vi "Finish.vi"   [LabVIEW 2012]
doc: "This VI is called just before exiting. It is expected to close I/O refnum, save collected data, etc."
uses:
  <vilib>/Rock Robotics/WPI/Compressor/WPI_CompressorGetSetRefNum.vi
  <vilib>/Rock Robotics/WPI/Joystick/WPI_JoystickGetSetRefNum.vi
  <vilib>/Rock Robotics/WPI/RobotDrive/WPI_RobotDriveGetSetRefNum.vi
types:
  T1 = typedef "WPI_JoystickDevRef.ctl" = cluster{"Device":T2}
  T2 = typedef "WPI_JoystickDeviceEnum.ctl" = enum16{"USB 1", "USB 2", "USB 3", "USB 4", "Kinect 1", "Kinect 2"}
  T3 = typedef "WPI_RobotDriveDevRef.ctl" = cluster{"DevStatus":errorcluster, "Motors[]":T4[], "Square Inputs":bool, "Max Output":dbl, "Isochronous":bool}
  T4 = typedef "WPI_MotorControlDeviceRef.ctl" = cluster{"DeviceStatus":errorcluster, "Type":enum16{"PWM", "CAN"}, "PWM":cluster{"Digital Module":T5, "PWM Channel":T6, "DeadBand":T7}, "CAN":cluster{"Device Number":u8, "Control Mode":T8, "Semaphore":T9, "Max Vout":dbl}, "Invert":bool, "TransformRef":T10, "InvTransformRef":T10}
  T5 = typedef "FPGA_TypedefDigitalModule.ctl" = enum16{"Digital Module 1", "Digital Module 2"}
  T6 = typedef "FPGA_DIOPWMChannel.ctl" = enum8{"PWM 1", "PWM 2", "PWM 3", "PWM 4", "PWM 5", "PWM 6", "PWM 7", "PWM 8", "PWM 9", "PWM 10", "Invalid"}
  T7 = typedef "WPI_PWMDeadband.ctl" = cluster{"Name":string, "maxPositivePwm":i32, "minPositivePwm":i32, "centerPwm":i32, "maxNegativePwm":i32, "minNegativePwm":i32, "angularRange":u16}
  T8 = typedef "WPI_CANJaguar_ControlMode.ctl" = enum8{"Percent VBus", "Current", "Speed", "Position", "Voltage"}
  T9 = typedef "Semaphore RefNum" = refnum<k1>
  T10 = typedef "WPI_PWMTransform_ConPane.ctl" = refnum<vi>
  T11 = typedef "WPI_CameraDevRef.ctl" = cluster{"Camera Address":string, "CameraStatus":errorcluster, "Acquire Image Notifier":refnum<notifier>}
  T12 = typedef "WPI_DigitalInputDevRef.ctl" = cluster{"DevStatus":errorcluster, "DIO Channel":T13, "Digital Module":T5}
  T13 = typedef "FPGA_DIOChannel.ctl" = enum8{"DIO 1", "DIO 2", "DIO 3", "DIO 4", "DIO 5", "DIO 6", "DIO 7", "DIO 8", "DIO 9", "DIO 10", "DIO 11", "DIO 12", "DIO 13", "DIO 14", "Invalid"}
  T14 = typedef "WPI_SolenoidDevRef.ctl" = cluster{"DevStatus":errorcluster, "Solenoid Module":T15, "Forward Solenoid Channel":T16, "Reverse Solenoid Channel":T16}
  T15 = typedef "FPGA_TypedefSolenoidModule.ctl" = enum16{"Solenoid Module 1", "Solenoid Module 2"}
  T16 = typedef "WPI_SolenoidChannel.ctl" = enum8{"Solenoid 1", "Solenoid 2", "Solenoid 3", "Solenoid 4", "Solenoid 5", "Solenoid 6", "Solenoid 7", "Solenoid 8", "Invalid"}
  T17 = typedef "WPI_CompressorDevRef.ctl" = cluster{"DevStatus":errorcluster, "DigitalInputDevRef":T12, "RelayDevRef":T18}
  T18 = typedef "WPI_RelayDevRef.ctl" = cluster{"DevStatus":errorcluster, "Relay Channel":T19, "Digital Module":T5, "Relay Direction":T20}
  T19 = typedef "FPGA_DIORelayChannel.ctl" = enum8{"Relay 1", "Relay 2", "Relay 3", "Relay 4", "Relay 5", "Relay 6", "Relay 7", "Relay 8", "Invalid"}
  T20 = typedef "WPI_RelayDirection.ctl" = enum16{"Both directions", "Forward only", "Reverse only"}
  T21 = typedef "WPI_EncoderDevRef.ctl" = cluster{"DevStatus":errorcluster, "EncoderIndex":T22, "CounterIndex":T23, "DistancePerCount":dbl, "Decoding Type":T24}
  T22 = typedef "FPGA_EncoderIdx.ctl" = enum8{"Enc 0", "Enc 1", "Enc 2", "Enc 3", "Invalid"}
  T23 = typedef "FPGA_CounterCtrSystemIndex.ctl" = enum8{"Ctr 0", "Ctr 1", "Ctr 2", "Ctr 3", "Ctr 4", "Ctr 5", "Ctr 6", "Ctr 7", "Invalid"}
  T24 = typedef "WPI_EncoderType.ctl" = enum16{"1x", "2x", "4x"}
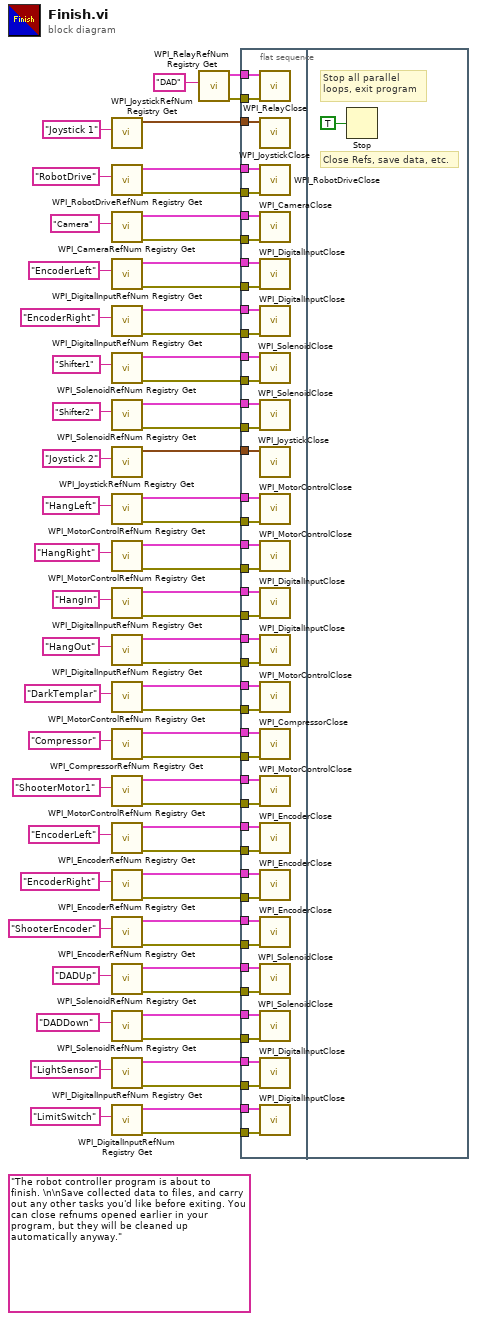
[diagram p0: block diagram]
diagram:
  (unwired) "The robot controller program is about to finish. \n\nSave collected data to files, and carry out any other tasks you'd like before exiting. You can close refnums opened earlier in your program, but they will be cleaned up automatically anyway."
  n1 = call <vilib>:"WPI_JoystickRefNum Registry Get.vi"("refnum name"="Joystick 1") -> ("JoystickDevRef"=w64:T1)  [unwired: 1 in, 9 out]
  n2 = call <vilib>:"WPI_RobotDriveRefNum Registry Get.vi"("refnum name"="RobotDrive") -> ("error out"=w61:errorcluster, "RobotDriveDevRef"=w65:T3)  [unwired: 1 in, 8 out]
  n3 = call <vilib>:"WPI_CameraRefNum Registry Get.vi"("refnum name"="Camera") -> ("error out"=w60:errorcluster, "CameraDevRef"=w63:T11)  [unwired: 1 in, 8 out]
  n4 = call <vilib>:"WPI_DigitalInputRefNum Registry Get.vi"("refnum name"="EncoderLeft") -> ("error out"=w54:errorcluster, "DigitalInputDevRef"=w55:T12)  [unwired: 9 in]
  n5 = call <vilib>:"WPI_DigitalInputRefNum Registry Get.vi"("refnum name"="EncoderRight") -> ("error out"=w53:errorcluster, "DigitalInputDevRef"=w48:T12)  [unwired: 9 in]
  n6 = call <vilib>:"WPI_SolenoidRefNum Registry Get.vi"("refnum name"="Shifter1") -> ("error out"=w51:errorcluster, "SolenoidDevRef"=w52:T14)  [unwired: 9 in]
  n7 = call <vilib>:"WPI_SolenoidRefNum Registry Get.vi"("refnum name"="Shifter2") -> ("error out"=w49:errorcluster, "SolenoidDevRef"=w50:T14)  [unwired: 9 in]
  n8 = call <vilib>:"WPI_JoystickRefNum Registry Get.vi"("refnum name"="Joystick 2") -> ("JoystickDevRef"=w47:T1)  [unwired: 1 in, 9 out]
  n9 = call <vilib>:"WPI_MotorControlRefNum Registry Get.vi"("refnum name"="HangLeft") -> ("error out"=w43:errorcluster, "MotorControlDevRef"=w44:T4)  [unwired: 9 in]
  n10 = call <vilib>:"WPI_MotorControlRefNum Registry Get.vi"("refnum name"="HangRight") -> ("error out"=w42:errorcluster, "MotorControlDevRef"=w41:T4)  [unwired: 9 in]
  n11 = call <vilib>:"WPI_DigitalInputRefNum Registry Get.vi"("refnum name"="HangIn") -> ("error out"=w38:errorcluster, "DigitalInputDevRef"=w39:T12)  [unwired: 9 in]
  n12 = call <vilib>:"WPI_DigitalInputRefNum Registry Get.vi"("refnum name"="HangOut") -> ("error out"=w35:errorcluster, "DigitalInputDevRef"=w34:T12)  [unwired: 9 in]
  n13 = call <vilib>:"WPI_MotorControlRefNum Registry Get.vi"("refnum name"="DarkTemplar") -> ("error out"=w31:errorcluster, "MotorControlDevRef"=w32:T4)  [unwired: 9 in]
  n14 = call <vilib>:"WPI_CompressorRefNum Registry Get.vi"("refnum name"="Compressor") -> ("error out"=w28:errorcluster, "CompressorDevRef"=w29:T17)  [unwired: 9 in]
  n15 = call <vilib>:"WPI_MotorControlRefNum Registry Get.vi"("refnum name"="ShooterMotor1") -> ("error out"=w27:errorcluster, "MotorControlDevRef"=w26:T4)  [unwired: 9 in]
  n16 = call <vilib>:"WPI_EncoderRefNum Registry Get.vi"("refnum name"="EncoderLeft") -> ("error out"=w22:errorcluster, "EncoderDevRef"=w23:T21)  [unwired: 9 in]
  n17 = call <vilib>:"WPI_EncoderRefNum Registry Get.vi"("refnum name"="EncoderRight") -> ("error out"=w21:errorcluster, "EncoderDevRef"=w20:T21)  [unwired: 9 in]
  n18 = call <vilib>:"WPI_EncoderRefNum Registry Get.vi"("refnum name"="ShooterEncoder") -> ("error out"=w16:errorcluster, "EncoderDevRef"=w17:T21)  [unwired: 9 in]
  n19 = call <vilib>:"WPI_SolenoidRefNum Registry Get.vi"("refnum name"="DADUp") -> ("error out"=w13:errorcluster, "SolenoidDevRef"=w14:T14)  [unwired: 9 in]
  n20 = call <vilib>:"WPI_SolenoidRefNum Registry Get.vi"("refnum name"="DADDown") -> ("error out"=w12:errorcluster, "SolenoidDevRef"=w11:T14)  [unwired: 9 in]
  n21 = call <vilib>:"WPI_DigitalInputRefNum Registry Get.vi"("refnum name"="LightSensor") -> ("error out"=w5:errorcluster, "DigitalInputDevRef"=w6:T12)  [unwired: 9 in]
  n22 = call <vilib>:"WPI_DigitalInputRefNum Registry Get.vi"("refnum name"="LimitSwitch") -> ("error out"=w2:errorcluster, "DigitalInputDevRef"=w1:T12)  [unwired: 9 in]
  n23 = call <vilib>:"WPI_RelayRefNum Registry Get.vi"("refnum name"="DAD") -> ("error out"=w7:errorcluster, "RelayDevRef"=w8:T18)  [unwired: 9 in]
  n24 = flat-sequence {
    tunnel: w65 -> [w111]
    tunnel: w64 -> [w110]
    tunnel: w63 -> [w109]
    tunnel: w61 -> [w108]
    tunnel: w60 -> [w107]
    tunnel: w55 -> [w106]
    tunnel: w54 -> [w105]
    tunnel: w53 -> [w104]
    tunnel: w52 -> [w103]
    tunnel: w51 -> [w102]
    tunnel: w50 -> [w101]
    tunnel: w49 -> [w100]
    tunnel: w48 -> [w99]
    tunnel: w47 -> [w98]
    tunnel: w44 -> [w97]
    tunnel: w43 -> [w96]
    tunnel: w41 -> [w94]
    tunnel: w42 -> [w95]
    tunnel: w38 -> [w92]
    tunnel: w39 -> [w93]
    tunnel: w35 -> [w91]
    tunnel: w34 -> [w90]
    tunnel: w32 -> [w89]
    tunnel: w31 -> [w88]
    tunnel: w29 -> [w87]
    tunnel: w28 -> [w86]
    tunnel: w26 -> [w84]
    tunnel: w27 -> [w85]
    tunnel: w23 -> [w83]
    tunnel: w22 -> [w82]
    tunnel: w20 -> [w80]
    tunnel: w21 -> [w81]
    tunnel: w17 -> [w79]
    tunnel: w16 -> [w78]
    tunnel: w14 -> [w77]
    tunnel: w13 -> [w76]
    tunnel: w11 -> [w74]
    tunnel: w12 -> [w75]
    tunnel: w8 -> [w73]
    tunnel: w7 -> [w72]
    tunnel: w5 -> [w70]
    tunnel: w6 -> [w71]
    tunnel: w2 -> [w69]
    tunnel: w1 -> [w68]
    frame #0 {
      n25 = call <vilib>:"WPI_RelayClose.vi"("error in (no error)"=w72, "RelayDevRef"=w73) -> ()  [unwired: 9 in, 1 out]
      n26 = call <vilib>:"WPI_JoystickClose.vi"("JoystickDevRef"=w110) -> ()  [unwired: 11 out]
      n27 = call <vilib>:"WPI_RobotDriveClose.vi"("error in (no error)"=w108, "RobotDriveDevRef"=w111) -> ()  [unwired: 10 out]
      n28 = call <vilib>:"WPI_CameraClose.vi"("error in (no error)"=w107, "CameraDevRef"=w109) -> ()  [unwired: 10 out]
      n29 = call <vilib>:"WPI_DigitalInputClose.vi"("error in (no error)"=w105, "DigitalInputDevRef"=w106) -> ()  [unwired: 9 in, 1 out]
      n30 = call <vilib>:"WPI_DigitalInputClose.vi"("error in (no error)"=w104, "DigitalInputDevRef"=w99) -> ()  [unwired: 9 in, 1 out]
      n31 = call <vilib>:"WPI_SolenoidClose.vi"("error in (no error)"=w102, "SolenoidDevRef"=w103) -> ()  [unwired: 9 in, 1 out]
      n32 = call <vilib>:"WPI_SolenoidClose.vi"("error in (no error)"=w100, "SolenoidDevRef"=w101) -> ()  [unwired: 9 in, 1 out]
      n33 = call <vilib>:"WPI_JoystickClose.vi"("JoystickDevRef"=w98) -> ()  [unwired: 11 out]
      n34 = call <vilib>:"WPI_MotorControlClose.vi"("error in (no error)"=w96, "MotorControlDevRef"=w97) -> ()  [unwired: 9 in, 1 out]
      n35 = call <vilib>:"WPI_MotorControlClose.vi"("error in (no error)"=w95, "MotorControlDevRef"=w94) -> ()  [unwired: 9 in, 1 out]
      n36 = call <vilib>:"WPI_DigitalInputClose.vi"("error in (no error)"=w92, "DigitalInputDevRef"=w93) -> ()  [unwired: 9 in, 1 out]
      n37 = call <vilib>:"WPI_DigitalInputClose.vi"("error in (no error)"=w91, "DigitalInputDevRef"=w90) -> ()  [unwired: 9 in, 1 out]
      n38 = call <vilib>:"WPI_MotorControlClose.vi"("error in (no error)"=w88, "MotorControlDevRef"=w89) -> ()  [unwired: 9 in, 1 out]
      n39 = call <vilib>:"WPI_CompressorClose.vi"("error in (no error)"=w86, "CompressorDevRef"=w87) -> ()  [unwired: 9 in, 1 out]
      n40 = call <vilib>:"WPI_MotorControlClose.vi"("error in (no error)"=w85, "MotorControlDevRef"=w84) -> ()  [unwired: 9 in, 1 out]
      n41 = call <vilib>:"WPI_EncoderClose.vi"("error in (no error)"=w82, "EncoderDevRef"=w83) -> ()  [unwired: 9 in, 1 out]
      n42 = call <vilib>:"WPI_EncoderClose.vi"("error in (no error)"=w81, "EncoderDevRef"=w80) -> ()  [unwired: 9 in, 1 out]
      n43 = call <vilib>:"WPI_EncoderClose.vi"("error in (no error)"=w78, "EncoderDevRef"=w79) -> ()  [unwired: 9 in, 1 out]
      n44 = call <vilib>:"WPI_SolenoidClose.vi"("error in (no error)"=w76, "SolenoidDevRef"=w77) -> ()  [unwired: 9 in, 1 out]
      n45 = call <vilib>:"WPI_SolenoidClose.vi"("error in (no error)"=w75, "SolenoidDevRef"=w74) -> ()  [unwired: 9 in, 1 out]
      n46 = call <vilib>:"WPI_DigitalInputClose.vi"("error in (no error)"=w70, "DigitalInputDevRef"=w71) -> ()  [unwired: 9 in, 1 out]
      n47 = call <vilib>:"WPI_DigitalInputClose.vi"("error in (no error)"=w69, "DigitalInputDevRef"=w68) -> ()  [unwired: 9 in, 1 out]
    }
    frame #1 {
      # "Close Refs, save data, etc."
      # "Stop all parallel\nloops, exit program"
      n48 = Stop(stop? (T)=TRUE ("Quit")) -> ()
    }
  }
